vi "Splash Screen State FGV.vi"(7 "Operation":enum16{"GET", "SET"}(ring), 8 "Error In":errorcluster, 11 "Close Splash Screen":bool) -> (0 "Error Out":errorcluster, 3 "Close Splash Screen Out":bool)   [LabVIEW 2014]
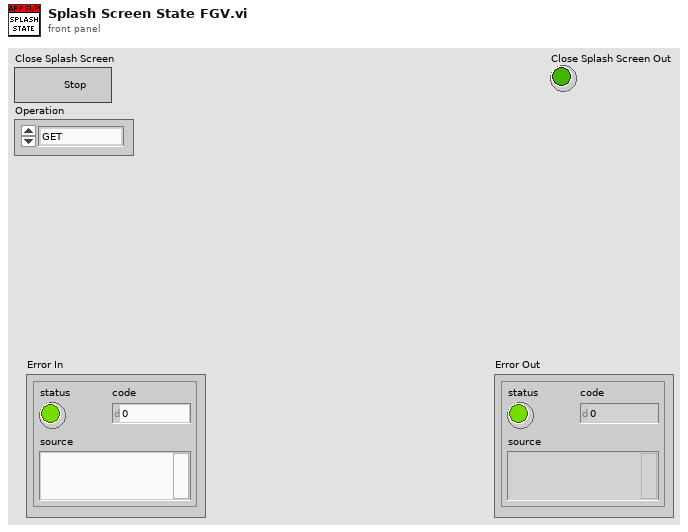
[diagram p1: front panel]
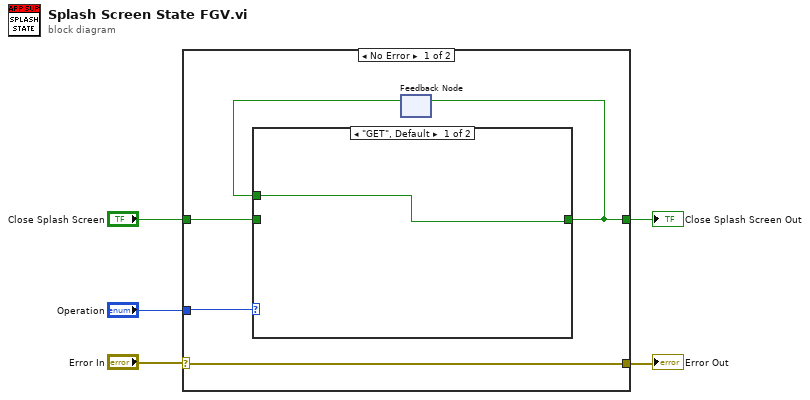
[diagram p0: block diagram]
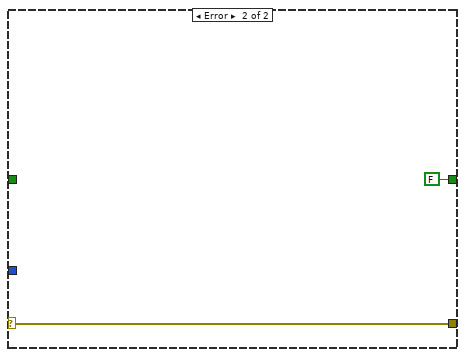
[diagram p3: hidden frame]
diagram:
  n1 = case shown="No Error" "Error In" {
    selector: "Error In" -> [w6 w13]
    tunnel: "Operation" -> [w10 _]
    tunnel: "Close Splash Screen" -> [w9 _]
    tunnel: [w8 FALSE ("Close Splash Screen")] -> w3
    tunnel: [w6 w13] -> w1
    frame No Error {
      n2 = feedback #1() -> (w7:bool)  [unwired: 1 in]
      n3 = case shown="\"GET\", Default" w10 {
        tunnel: w9 -> [_ w12]
        tunnel: [w11 w12] -> w8
        tunnel: w7 -> [w11 _]
        frame "GET", Default {
        }
        frame "SET" {
        }
      }
      n4 = feedback-in #1(w8) -> ()
    }
    frame Error {
    }
  }
  "Close Splash Screen Out" <- w3
  "Error Out" <- w1
